vi "ejer7.vi"() -> ()   [LabVIEW 2014]
uses:
  TAREA PARTE II/ejer7.ctl
panel:
  in  "Selector":string(combo)
  in  "Apagar el Medidor":bool
  in  "?":bool
  out "Lectura":string
  out "Medidor":dbl(knob) scale=0.0..15.0
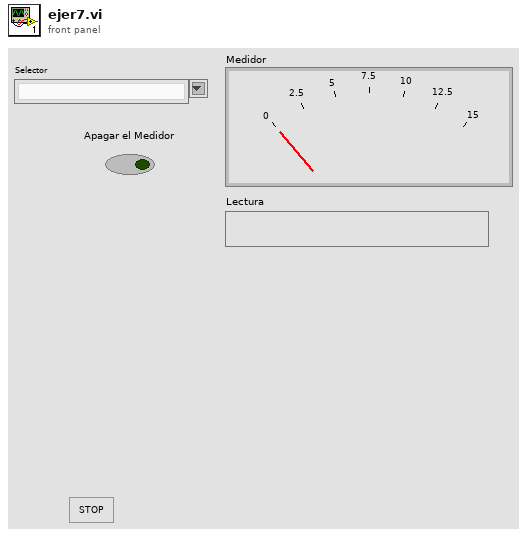
[diagram p1: front panel]
types:
  T1 = typedef "ejer7.ctl" = string
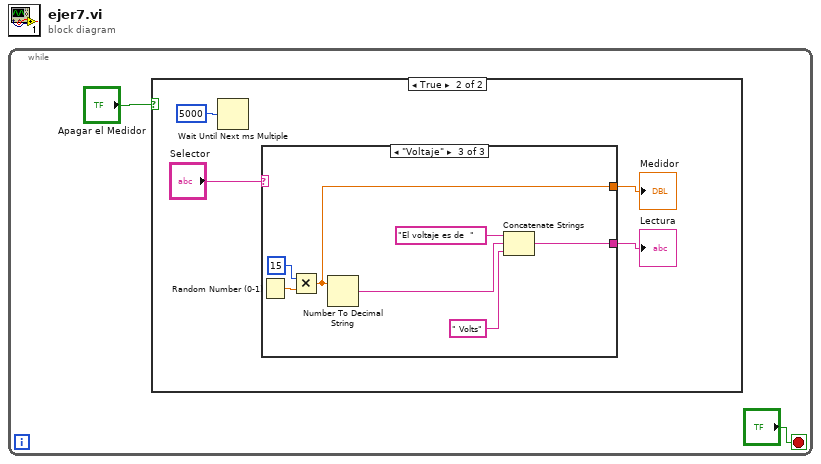
[diagram p0: block diagram]
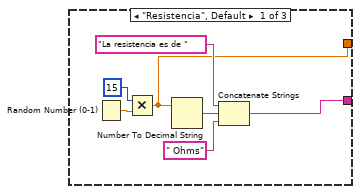
[diagram p3: hidden frame]
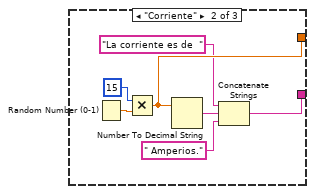
[diagram p4: hidden frame]
diagram:
  n1 = while {
    stop <- "?" stop-if-true
    n2 = case shown="True" "Apagar el Medidor" {
      frame False {
      }
      frame True {
        n3 = Wait Until Next ms Multiple(millisecond multiple=5000) -> ()  [unwired: 1 out]
        n4 = case shown="\"Voltaje\"" "Selector" {
          tunnel: [w8 w14 w21] -> w6
          tunnel: [w9 w20 w23] -> w4
          frame "Resistencia", Default {
            n5 = Random Number (0-1)() -> (number: 0 to 1=w11:dbl)
            n6 = Multiply(x=15 ("Numeric"), y=w11) -> (x*y=w9:dbl)
            n7 = Number To Decimal String(number=w9) -> (decimal integer string=w12:string)  [unwired: 1 in]
            n8 = Concatenate Strings("La resistencia es de ", w12, T1 " Ohms") -> (w8:string)
          }
          frame "Corriente" {
            n9 = Random Number (0-1)() -> (number: 0 to 1=w18:dbl)
            n10 = Multiply(x=15 ("Numeric"), y=w18) -> (x*y=w20:dbl)
            n11 = Number To Decimal String(number=w20) -> (decimal integer string=w16:string)  [unwired: 1 in]
            n12 = Concatenate Strings("La corriente es de  ", w16, " Amperios.") -> (w14:string)
          }
          frame "Voltaje" {
            n13 = Random Number (0-1)() -> (number: 0 to 1=w25:dbl)
            n14 = Multiply(x=15 ("Numeric"), y=w25) -> (x*y=w23:dbl)
            n15 = Number To Decimal String(number=w23) -> (decimal integer string=w26:string)  [unwired: 1 in]
            n16 = Concatenate Strings "Concatenate Strings"("El voltaje es de  ", w26, " Volts") -> (w21:string)
          }
        }
        "Medidor" <- w4
        "Lectura" <- w6
      }
    }
  }
